vi "State_Modelling_2_state_sol..vi"() -> ()   [LabVIEW 2019]
uses:
  <vilib>/addons/Control Design/_Model Construction/NI_LinSys_Model Creation.lvlib
  <vilib>/addons/Control Design/_Model Construction/Model Creation.llb/Model Creation SubVI/cd_Create State Space Model.vi
  <vilib>/addons/Control Design/_State-Space Analysis/NI_CD_State-Space Analysis.lvlib
  <vilib>/addons/Control Design/_Utility/NI_CD_Model Viewer.lvlib
  <vilib>/addons/Control Design/_Utility/Model Viewer.llb/Model Viewer SubVI/cd_Draw State-Space Equation (SS).vi
  <vilib>/addons/Control Design/_Dynamic Analysis/NI_CD_Dynamic Analysis.lvlib
  <vilib>/addons/Control Design/_Dynamic Analysis/Dynamic Analysis.llb/Dynamic Analysis subVI/cd_Pole-Zero Map (State-Space).vi
  <vilib>/addons/Control Design/_Time Response Analysis/NI_CD_Time Response.lvlib
  <vilib>/addons/Control Design/_Time Response Analysis/Time Response.llb/Time Response subVI/cd_Initial Response (State-Space).vi
  <vilib>/addons/Control Design/_State Feedback Control/NI_CD_State Feedback Control.lvlib
  <vilib>/Analysis/NI_AALBase.lvlib
  <vilib>/Analysis/baseanly.llb/Real A x B.vi
  <vilib>/Analysis/Matrix/NI_Matrix.lvlib
  <vilib>/Analysis/Matrix/Numeric/Subtract/Subtract - RM,RM.vi
  <vilib>/addons/Control Design/_Dynamic Analysis/Dynamic Analysis.llb/Dynamic Analysis subVI/cd_Root Locus (State-Space).vi
panel:
  in  "Compenstaed Root Locus Gain":dbl[](array[numeric])=[1e-18] format="%.2f"
  out "Compensated Root Locus":cluster{dbl[], dbl[]}[](graph)=[{[-5.0, -5.0], [1.0323827311807139e-07, -1.0323827311807139e-07]}, {[-4.999999999999999, -4.999999999999999], [1.0323827311807139e-07, -1.0323827311807139e-07]}, {[], []}, {[-4.999999999999999], [0.0]}, {array[592 elements], [1.0323827311807139e-07, 5.960464477539063e-08, 5.960464477539063e-08, 5.960464477539063e-08, 5.960464477539063e-08, 5.960464477539063e-08, 5.960464477539063e-08, 5.960464477539063e-08, 5.960464477539063e-08, 5.960464477539063e-08, 5.960464477539063e-08, 0.0, 0.0, 0.0, 0.0, 0.0, 0.0, 0.0, 0.0, 0.0, 0.0, 0.0, 0.0, 0.0, 0.0, 0.0, 0.0, 0.0, 0.0, 0.0, 0.0, 0.0, 0.0, 0.0, 0.0, 0.0, 0.0, 0.0, 0.0, 0.0, 0.0, 0.0, 0.0, 0.0, 0.0, 0.0, 0.0, 0.0, 0.0, 0.0, 0.0, 0.0, 0.0, 0.0, 0.0, 0.0, 0.0, 0.0, 0.0, 0.0, 0.0, 0.0, 0.0, 0.0, 0.0, 0.0, 0.0, 0.0, 0.0, 0.0, 0.0, 0.0, 0.0, 0.0, 0.0, 0.0, 0.0, 0.0, 0.0, 0.0, 0.0, 0.0, 0.0, 0.0, 0.0, 0.0, 0.0, 0.0, 0.0, 0.0, 0.0, 0.0, 0.0, 0.0, 0.0, 0.0, 0.0, 0.0, 0.0, 0.0, 0.0, 0.0, 0.0, 0.0, 0.0, 0.0, 0.0, 0.0, 0.0, 0.0, 0.0, 0.0, 0.0, 0.0, 0.0, 0.0, 0.0, 0.0, 0.0, 0.0, 0.0, 0.0, 0.0, 0.0, 0.0, 0.0, 0.0, 0.0, 0.0, 0.0, 0.0, 0.0, 0.0, 0.0, 0.0, 0.0, 0.0, 0.0, 0.0, 0.0, 0.0, 0.0, 0.0, 0.0, 0.0, 0.0, 0.0, 0.0, 0.0, 0.0, 0.0, 0.0, 0.0, 0.0, 0.0, 0.0, 0.0, 0.0, 0.0, 0.0, 0.0, 0.0, 0.0, 0.0, 0.0, 0.0, 0.0, 0.0, 0.0, 0.0, 0.0, 0.0, 0.0, 0.0, 0.0, 0.0, 0.0, 0.0, 0.0, 0.0, 0.0, 0.0, 0.0, 0.0, 0.0, 0.0, 0.0, 0.0, 0.0, 0.0, 0.0, 0.0, 0.0, 0.0, 0.0, 0.0, 0.0, 0.0, 0.0, 0.0, 0.0, 0.0, 0.0, 0.0, 0.0, 0.0, 0.0, 0.0, 0.0, 0.0, 0.0, 0.0, 0.0, 0.0, 0.0, 0.0, 0.0, 0.0, 0.0, 0.0, 0.0, 0.0, 0.0, 0.0, 0.0, 0.0, 0.0, 0.0, 0.0, 0.0, 0.0, 0.0, 0.0, 0.0, 0.0, 0.0, 0.0, 0.0, 0.0, 0.0, 0.0, 0.0, 0.0, 0.0, 0.0, 0.0, 0.0, 0.0, 0.0, 0.0, 0.0, 0.0, 0.0, 0.0, 0.0, 0.0, 0.0, 0.0, 0.0, 0.0, 0.0, 0.0, 0.0, 0.0, 0.0, 0.0, 0.0, 0.0, 0.0, 0.0, 0.0, 0.0, 0.0, 0.0, 0.0, 0.0, 0.0, 0.0, 0.0, 0.0, 0.0, 0.0, 0.0, 0.0, 0.0, 0.0, 0.0, 0.0, 0.0, 0.0, 0.0, 0.0, 0.0, 0.0, 0.0, 0.0, 0.0, 0.0, 0.0, 0.0, 0.0, 0.0, 0.0, 0.0, 0.0, 0.0, 0.0, 0.0, 0.0, 0.0, 0.0, 0.0, 0.0, 0.0, 0.0, 0.0, 0.0, 0.0, 0.0, 0.0, 0.0, 0.0, 0.0, nan, nan, nan, nan, nan, nan, nan, nan, nan, nan, nan, nan, nan, nan, nan, nan, nan, nan, nan, nan, nan, nan, nan, nan, nan, nan, nan, nan, nan, nan, nan, nan, nan, nan, nan, nan, nan, nan, nan, nan, nan, nan, nan, nan, nan, nan, nan, nan, nan, nan, nan, nan, nan, nan, nan, nan, nan, nan, nan, nan, nan, nan, nan, nan, nan, nan, nan, nan, nan, nan, nan, nan, nan, nan, nan, nan, nan, nan, nan, nan, nan, nan, nan, nan, nan, nan, nan, nan, nan, nan, nan, nan, nan, nan, nan, nan, nan, nan, nan, nan, nan, nan, nan, nan, nan, nan, nan, nan, nan, nan, nan, nan, nan, nan, nan, nan, nan, nan, nan, nan, nan, nan, nan, nan, nan, nan, nan, nan, nan, nan, nan, nan, nan, nan, nan, nan, nan, nan, nan, nan, nan, nan, nan, nan, nan, nan, nan, nan, nan, nan, nan, nan, nan, nan, nan, nan, nan, nan, nan, nan, nan, nan, nan, nan, nan, nan, nan, nan, nan, nan, nan, nan, nan, nan, nan, nan, nan, nan, nan, nan, nan, nan, nan, nan, nan, nan, nan, nan, nan, nan, nan, nan, nan, nan, nan, nan, nan, nan, nan, nan, nan, nan, nan, nan, nan, nan, nan, nan, nan, nan, nan, nan, nan, nan, nan, nan, nan, nan, nan, nan, nan, nan, nan, nan, nan, nan, nan, nan, nan, nan, nan, nan, nan, nan, nan, nan, nan, nan, nan, nan, nan, nan, nan, nan, nan, nan, nan, nan, nan, nan, nan, nan, nan, nan, nan, nan, nan, nan, nan, nan, nan, nan, nan, nan, nan, nan, nan, nan, nan]}, {array[592 elements], [-1.0323827311807139e-07, -5.960464477539063e-08, -5.960464477539063e-08, -5.960464477539063e-08, -5.960464477539063e-08, -5.960464477539063e-08, -5.960464477539063e-08, -5.960464477539063e-08, -5.960464477539063e-08, -5.960464477539063e-08, -5.960464477539063e-08, 0.0, 0.0, 0.0, 0.0, 0.0, 0.0, 0.0, 0.0, 0.0, 0.0, 0.0, 0.0, 0.0, 0.0, 0.0, 0.0, 0.0, 0.0, 0.0, 0.0, 0.0, 0.0, 0.0, 0.0, 0.0, 0.0, 0.0, 0.0, 0.0, 0.0, 0.0, 0.0, 0.0, 0.0, 0.0, 0.0, 0.0, 0.0, 0.0, 0.0, 0.0, 0.0, 0.0, 0.0, 0.0, 0.0, 0.0, 0.0, 0.0, 0.0, 0.0, 0.0, 0.0, 0.0, 0.0, 0.0, 0.0, 0.0, 0.0, 0.0, 0.0, 0.0, 0.0, 0.0, 0.0, 0.0, 0.0, 0.0, 0.0, 0.0, 0.0, 0.0, 0.0, 0.0, 0.0, 0.0, 0.0, 0.0, 0.0, 0.0, 0.0, 0.0, 0.0, 0.0, 0.0, 0.0, 0.0, 0.0, 0.0, 0.0, 0.0, 0.0, 0.0, 0.0, 0.0, 0.0, 0.0, 0.0, 0.0, 0.0, 0.0, 0.0, 0.0, 0.0, 0.0, 0.0, 0.0, 0.0, 0.0, 0.0, 0.0, 0.0, 0.0, 0.0, 0.0, 0.0, 0.0, 0.0, 0.0, 0.0, 0.0, 0.0, 0.0, 0.0, 0.0, 0.0, 0.0, 0.0, 0.0, 0.0, 0.0, 0.0, 0.0, 0.0, 0.0, 0.0, 0.0, 0.0, 0.0, 0.0, 0.0, 0.0, 0.0, 0.0, 0.0, 0.0, 0.0, 0.0, 0.0, 0.0, 0.0, 0.0, 0.0, 0.0, 0.0, 0.0, 0.0, 0.0, 0.0, 0.0, 0.0, 0.0, 0.0, 0.0, 0.0, 0.0, 0.0, 0.0, 0.0, 0.0, 0.0, 0.0, 0.0, 0.0, 0.0, 0.0, 0.0, 0.0, 0.0, 0.0, 0.0, 0.0, 0.0, 0.0, 0.0, 0.0, 0.0, 0.0, 0.0, 0.0, 0.0, 0.0, 0.0, 0.0, 0.0, 0.0, 0.0, 0.0, 0.0, 0.0, 0.0, 0.0, 0.0, 0.0, 0.0, 0.0, 0.0, 0.0, 0.0, 0.0, 0.0, 0.0, 0.0, 0.0, 0.0, 0.0, 0.0, 0.0, 0.0, 0.0, 0.0, 0.0, 0.0, 0.0, 0.0, 0.0, 0.0, 0.0, 0.0, 0.0, 0.0, 0.0, 0.0, 0.0, 0.0, 0.0, 0.0, 0.0, 0.0, 0.0, 0.0, 0.0, 0.0, 0.0, 0.0, 0.0, 0.0, 0.0, 0.0, 0.0, 0.0, 0.0, 0.0, 0.0, 0.0, 0.0, 0.0, 0.0, 0.0, 0.0, 0.0, 0.0, 0.0, 0.0, 0.0, 0.0, 0.0, 0.0, 0.0, 0.0, 0.0, 0.0, 0.0, 0.0, 0.0, 0.0, 0.0, 0.0, 0.0, 0.0, 0.0, 0.0, 0.0, 0.0, 0.0, 0.0, 0.0, 0.0, 0.0, 0.0, 0.0, 0.0, 0.0, 0.0, 0.0, 0.0, 0.0, 0.0, 0.0, 0.0, 0.0, 0.0, 0.0, 0.0, 0.0, 0.0, 0.0, 0.0, 0.0, 0.0, 0.0, 0.0, 0.0, 0.0, 0.0, 0.0, 0.0, 0.0, 0.0, 0.0, 0.0, 0.0, 0.0, 0.0, 0.0, 0.0, 0.0, 0.0, 0.0, 0.0, 0.0, 0.0, 0.0, 0.0, 0.0, 0.0, 0.0, 0.0, 0.0, 0.0, 0.0, 0.0, 0.0, 0.0, 0.0, 0.0, 0.0, 0.0, 0.0, 0.0, 0.0, 0.0, 0.0, 0.0, 0.0, 0.0, 0.0, 0.0, 0.0, 0.0, 0.0, 0.0, 0.0, 0.0, 0.0, 0.0, 0.0, 0.0, 0.0, 0.0, 0.0, 0.0, 0.0, 0.0, 0.0, 0.0, 0.0, 0.0, 0.0, 0.0, 0.0, 0.0, 0.0, 0.0, 0.0, 0.0, 0.0, 0.0, 0.0, 0.0, 0.0, 0.0, 0.0, 0.0, 0.0, 0.0, 0.0, 0.0, 0.0, 0.0, 0.0, 0.0, 0.0, 0.0, 0.0, 0.0, 0.0, 0.0, 0.0, 0.0, 0.0, 0.0, 0.0, 0.0, 0.0, 0.0, 0.0, 0.0, 0.0, 0.0, 0.0, 0.0, 0.0, 0.0, 0.0, 0.0, 0.0, 0.0, 0.0, 0.0, 0.0, nan, nan, nan, nan, nan, nan, nan, nan, nan, nan, nan, nan, nan, nan, nan, nan, nan, nan, nan, nan, nan, nan, nan, nan, nan, nan, nan, nan, nan, nan, nan, nan, nan, nan, nan, nan, nan, nan, nan, nan, nan, nan, nan, nan, nan, nan, nan, nan, nan, nan, nan, nan, nan, nan, nan, nan, nan, nan, nan, nan, nan, nan, nan, nan, nan, nan, nan, nan, nan, nan, nan, nan, nan, nan, nan, nan, nan, nan, nan, nan, nan, nan, nan, nan, nan, nan, nan, nan, nan, nan, nan, nan, nan, nan, nan, nan, nan, nan, nan, nan, nan, nan, nan, nan, nan, nan, nan, nan, nan, nan, nan, nan, nan, nan, nan, nan, nan, nan, nan, nan, nan, nan, nan, nan, nan, nan, nan, nan, nan, nan, nan, nan, nan, nan, nan, nan, nan, nan, nan, nan, nan, nan, nan, nan, nan, nan, nan, nan, nan, nan]}]
  out "Root Locus Graph":cluster{dbl[], dbl[]}[](graph)=[{[-1.1574212961095778e-15, -1.1574212961095778e-15], [-18.902124219251128, 18.902124219251128]}, {[-0.0, -0.0], [18.902124219251128, -18.902124219251128]}, {[], []}, {[0.0], [0.0]}, {array[574 elements], array[574 elements]}, {array[574 elements], array[574 elements]}]
  in  "Root Locus Gain":dbl[](array[numeric])=[0.0] format="%.2f"
  in  "Desired Poles":cdb[](array[numeric])=[-5.0+0.0i, -5.0+0.0i] format="%.2f"
  in  "D":dbl[][](array[numeric])=[[0.0]] format="%#.5g"
  in  "C":dbl[][](array[numeric])=[[1.0, 0.0]] format="%#.5g"
  in  "B":dbl[][](array[numeric])=[[0.0], [-36.421]] format="%#.5g"
  in  "A":dbl[][](array[numeric])=[[0.0, 1.0], [-357.2903, 0.0]] format="%#.5g"
  in  "Initial Conditions":dbl[](array[numeric])=[0.572, 0.0] format="%.3f"
  out "State Trajectory Graph Compensated":cluster{"time":dbl[], dbl[]}[](graph)=[{"time"=[0.0, 0.04000000000000001, 0.08000000000000002, 0.12000000000000002, 0.16000000000000003, 0.20000000000000004, 0.24000000000000005, 0.28, 0.32000000000000006, 0.3600000000000001, 0.4000000000000001, 0.44000000000000006, 0.4800000000000001, 0.5200000000000001, 0.56, 0.6000000000000001, 0.6400000000000001, 0.6800000000000002, 0.7200000000000002, 0.7600000000000001, 0.8000000000000002, 0.8400000000000002, 0.8800000000000001, 0.9200000000000002, 0.9600000000000002, 1.0000000000000002, 1.0400000000000003, 1.0800000000000003, 1.12, 1.1600000000000001, 1.2000000000000002, 1.2400000000000002, 1.2800000000000002, 1.3200000000000003, 1.3600000000000003, 1.4000000000000004, 1.4400000000000004, 1.4800000000000002, 1.5200000000000002, 1.5600000000000003, 1.6000000000000003], [0.572, 0.5619767889127265, 0.5367922928653396, 0.5022724093532525, 0.46262910145509073, 0.4208540807001293, 0.3790227962703144, 0.3385283120990366, 0.30026050156165074, 0.2647426993756922, 0.23223534603402665, 0.20281410106641523, 0.17642827555724877, 0.1529441522589557, 0.13217675212217317, 0.11391281242567214, 0.09792711883762648, 0.08399384583614819, 0.07189417850331574, 0.06142119120828786, 0.0523827272217794, 0.044602843694828566, 0.03792224749259751, 0.03219804025721003, 0.027303008809828617, 0.023124634100861116, 0.01956394406178582, 0.016534299514716293, 0.013960175102466216, 0.01177597693761364, 0.009924923715371986, 0.008358007132520252, 0.007033039625890542, 0.005913791932828125, 0.004969219199624306, 0.004172771874377408, 0.003501786075609926, 0.0029369472666753264, 0.002461820691381014, 0.0020624419901926214, 0.0017269616084421026]}, {"time"=[0.0, 0.04000000000000001, 0.08000000000000002, 0.12000000000000002, 0.16000000000000003, 0.20000000000000004, 0.24000000000000005, 0.28, 0.32000000000000006, 0.3600000000000001, 0.4000000000000001, 0.44000000000000006, 0.4800000000000001, 0.5200000000000001, 0.56, 0.6000000000000001, 0.6400000000000001, 0.6800000000000002, 0.7200000000000002, 0.7600000000000001, 0.8000000000000002, 0.8400000000000002, 0.8800000000000001, 0.9200000000000002, 0.9600000000000002, 1.0000000000000002, 1.0400000000000003, 1.0800000000000003, 1.12, 1.1600000000000001, 1.2000000000000002, 1.2400000000000002, 1.2800000000000002, 1.3200000000000003, 1.3600000000000003, 1.4000000000000004, 1.4400000000000004, 1.4800000000000002, 1.5200000000000002, 1.5600000000000003, 1.6000000000000003], [0.0, -0.46831399076060565, -0.7668461326647711, -0.9417607675373487, -1.028064669900202, -1.0521352017503238, -1.0336985352826762, -0.9873742436221906, -0.9238784663435413, -0.8509586765647255, -0.7741178201134225, -0.6971734724158027, -0.6226880313785255, -0.5522983276017848, -0.4869669815027436, -0.42717304659627087, -0.37305569081000595, -0.32452167709420926, -0.28132504631732275, -0.24312554853280632, -0.20953090888711776, -0.18012686876757705, -0.15449804534021222, -0.13224195105639847, -0.11297796748894612, -0.09635264208692143, -0.08204234606555352, -0.06975407607770943, -0.059224985283190076, -0.05022107811629353, -0.04253538735159428, -0.03598586404279558, -0.030413144328175358, -0.02567830707675374, -0.02166069907528547, -0.018255876950401186, -0.01537369496609238, -0.012936553436546098, -0.010877812357264961, -0.00914036791108095, -0.007675384926409356]}]
  out "Comp poles":cdb[](array[numeric])=[-4.999999999999999+9.425385918369788e-08i, -4.999999999999999-9.425385918369788e-08i] caption="Poles Compensated" format="%.4f"
  out "Pole-Zero Map Comp":cluster{dbl[], dbl[]}[](graph)=[{[-4.999999999999999, -4.999999999999999], [9.425385918369788e-08, -9.425385918369788e-08]}, {[], []}] caption="Pole-Zero Map Compensated"
  out "Actual Poles":cdb[](array[numeric])=[-4.999999999999999+9.425385918369788e-08i, -4.999999999999999-9.425385918369788e-08i] format="%.2f"
  out "Gain":dbl[][](array[numeric])=[[9.123590785535818, -0.27456687076137387]] format="%.2f"
  out "State Trajectory Graph":cluster{"time":dbl[], dbl[]}[](graph)
  out "Uncomp Poles":cdb[](array[numeric])=[0.0+18.902124219251128i, 0.0-18.902124219251128i] caption="Poles Uncompensated" format="%.4f"
  out "Pole-Zero Map":cluster{dbl[], dbl[]}[](graph)=[{[0.0, 0.0], [18.902124219251128, -18.902124219251128]}, {[], []}]
  out "Equation":picture
  out "Transformation Matrix (T)":dbl[][](array[numeric])=[[18.9285577897525, 0.0], [-0.0, 1.0013984444390887]] format="%.2f"
  in  "Form Type":u16(ring) items=["Modal"=0, "Companion"=5, "Controllability"=1, "Controller Companion"=2, "Observability"=3, "Observer Companion"=4]
  out "Is Controllable?":bool=TRUE
  out "Controllability Matrix":dbl[][](array[numeric])=[[0.0, -36.421], [-36.421, 0.0]] format="%.2f"
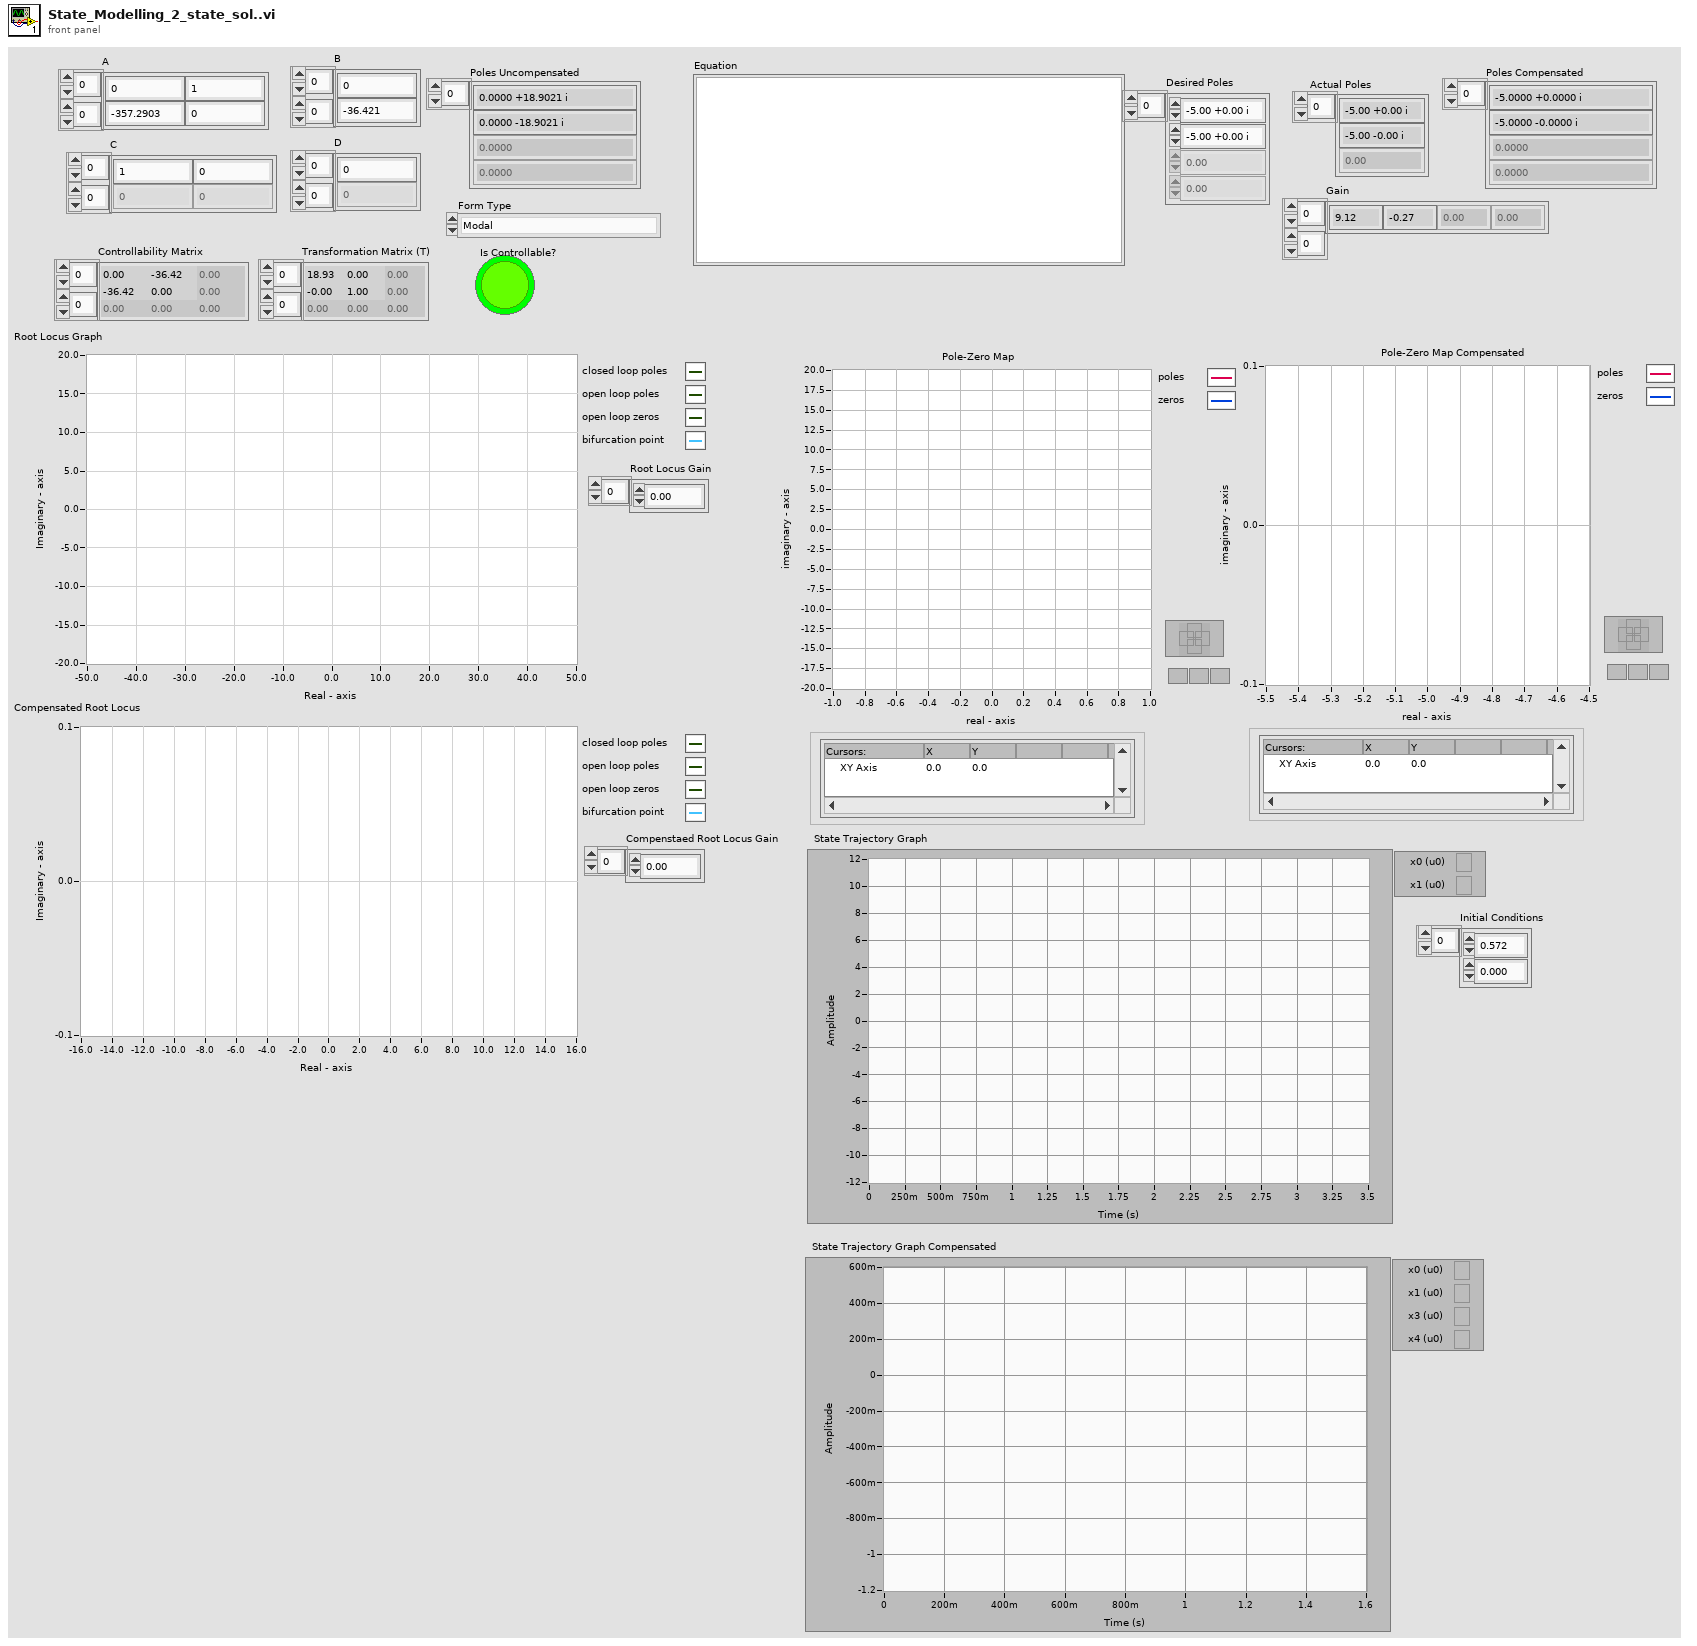
[diagram p1: front panel]
types:
  T1 = typedef "NI_LinSys_Model Typedefs.lvlib/CD State Space Model (MIMO).ctl" = cluster{"properties":T2, "A":dbl[][], "B":dbl[][], "C":dbl[][], "D":dbl[][], "StateNames":string[], "Transport Delay":dbl[][]}
  T2 = typedef "NI_LinSys_Model Typedefs.lvlib/CD General Elements.ctl" = cluster{"Model name":string, "Input names":string[], "Output names":string[], "Input Delays":dbl[], "Output Delays":dbl[], "Sampling Time":dbl, "Notes":string}
  T3 = typedef "NI_Matrix.lvlib/RealMatrix.ctl" = dbl[][]
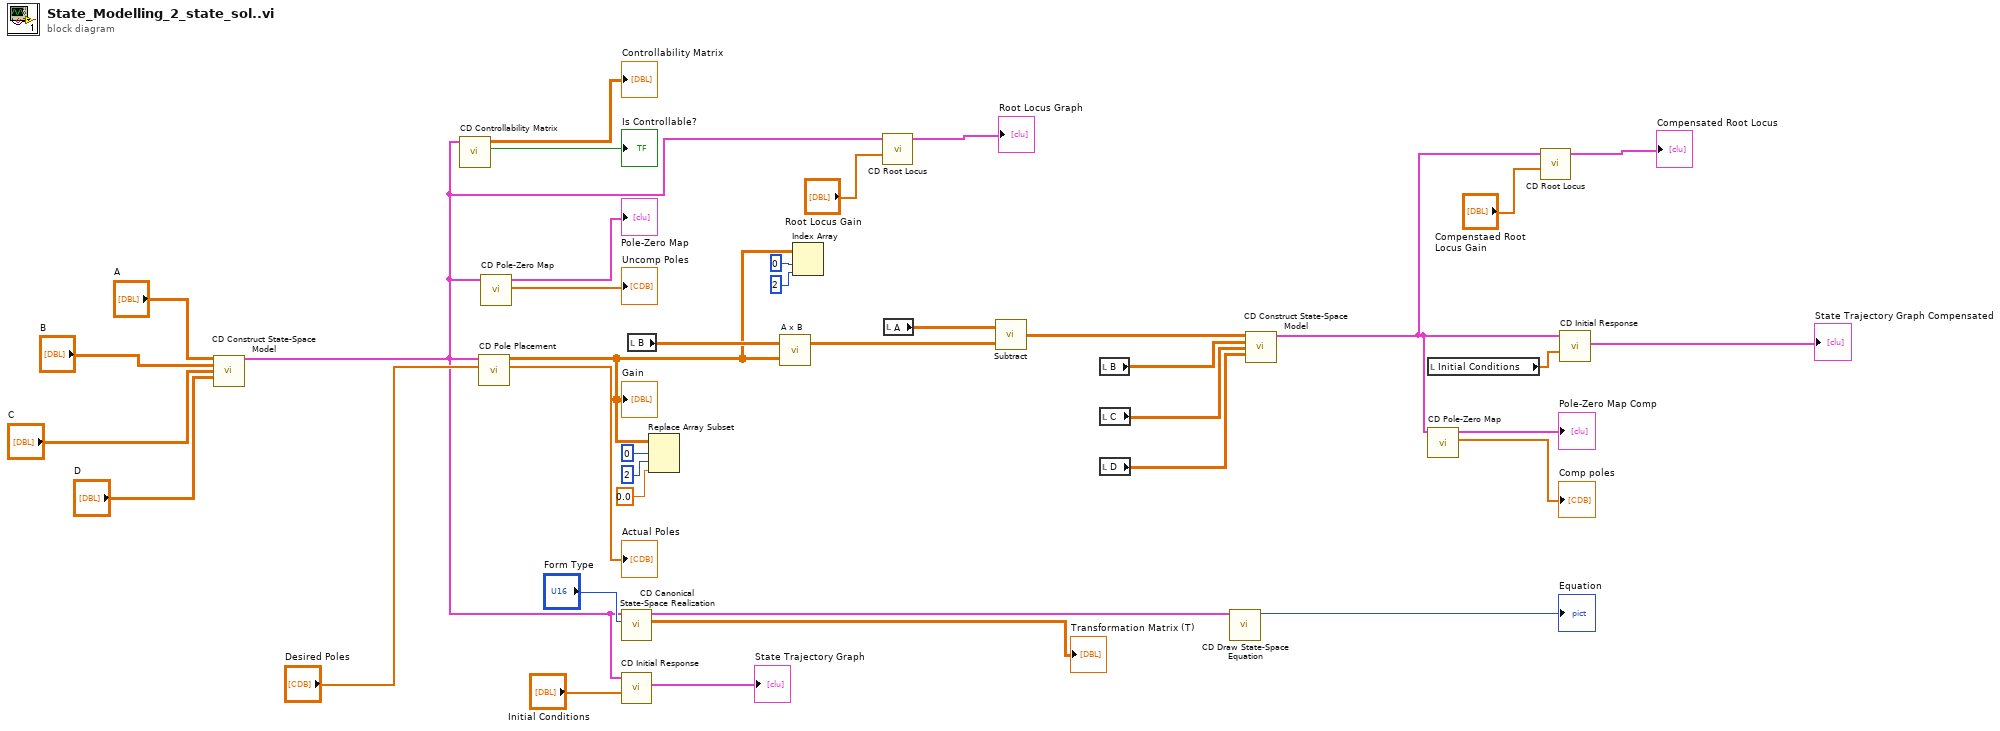
[diagram p0: block diagram]
diagram:
  n1 = call-poly <vilib>:"CD Construct State-Space Model.vi"("A"="A", "B"="B", "C"="C", "D"="D") -> ("State-Space Model"=w6:T1)  [unwired: 10 in, 1 out]
  n2 = call <vilib>:"CD Controllability Matrix.vi"("State-Space Model"=w6) -> ("Is Controllable?"=→"Is Controllable?":bool, "Controllability Matrix"=→"Controllability Matrix":dbl[][])  [unwired: 7 in, 2 out]
  n3 = call <vilib>:"CD Pole Placement.vi"("Poles"="Desired Poles", "State-Space Model"=w6) -> ("Actual Poles"=→"Actual Poles":cdb[], "Gain"=w8:dbl[][])  [unwired: 7 in, 1 out]
  "Gain" <- w8
  n4 = call-poly <vilib>:"CD Pole-Zero Map.vi"("State-Space Model"=w6) -> ("Poles"=→"Uncomp Poles":cdb[], "Pole-Zero Map"=→"Pole-Zero Map":cluster{dbl[], dbl[]}[])  [unwired: 7 in, 2 out]
  n5 = call <vilib>:"CD Canonical State-Space Realization.vi"("Form Type"="Form Type", "State-Space Model"=w6) -> ("Transformation Matrix (T)"=→"Transformation Matrix (T)":dbl[][], "Transformed Model"=w35:T1)  [unwired: 7 in, 1 out]
  n6 = call-poly <vilib>:"CD Initial Response.vi"("Initial Conditions"="Initial Conditions", "State-Space Model"=w6) -> ("State Trajectory Graph"=→"State Trajectory Graph":cluster{"time":dbl[], dbl[]}[])  [unwired: 6 in, 3 out]
  n7 = local read "B"() -> (w14:dbl[][])
  n8 = Replace Array Subset(array=w8, new element=0.0 ("new element/subarray"), index (row)=0, index (col)=2 ("disabled index (col)")) -> ()  [unwired: 1 out]
  n9 = call-poly <vilib>:"A x B.vi"("B"=w8, "A"=w14) -> ("A x B"=w28:T3)  [unwired: 1 out]
  n10 = Index Array(array=w8, index (row)=0, index (col)=2 ("disabled index (col)")) -> ()  [unwired: 1 out]
  n11 = call-poly <vilib>:"CD Root Locus.vi"("Gain"="Root Locus Gain", "State-Space Model"=w6) -> ("Root Locus Graph"=→"Root Locus Graph":cluster{dbl[], dbl[]}[])  [unwired: 6 in, 3 out]
  n12 = local read "A"() -> (w18:dbl[][])
  n13 = call-poly <vilib>:"Subtract.vi"("Real Matrix B"=w28, "Real Matrix A"=w18) -> ("A - B"=w26:T3)
  n14 = local read "B"() -> (w17:dbl[][])
  n15 = local read "C"() -> (w16:dbl[][])
  n16 = local read "D"() -> (w15:dbl[][])
  n17 = call-poly <vilib>:"CD Draw State-Space Equation.vi"("State-Space Model"=w35) -> ("Equation"=→"Equation":picture)  [unwired: 8 in, 2 out]
  n18 = call-poly <vilib>:"CD Construct State-Space Model.vi"("A"=w26, "B"=w17, "C"=w16, "D"=w15) -> ("State-Space Model"=w1:T1)  [unwired: 10 in, 1 out]
  n19 = local read "Initial Conditions"() -> (w19:dbl[])
  n20 = call-poly <vilib>:"CD Pole-Zero Map.vi"("State-Space Model"=w1) -> ("Poles"=→"Comp poles":cdb[], "Pole-Zero Map"=→"Pole-Zero Map Comp":cluster{dbl[], dbl[]}[])  [unwired: 7 in, 2 out]
  n21 = call-poly <vilib>:"CD Root Locus.vi"("Gain"="Compenstaed Root Locus Gain", "State-Space Model"=w1) -> ("Root Locus Graph"=→"Compensated Root Locus":cluster{dbl[], dbl[]}[])  [unwired: 6 in, 3 out]
  n22 = call-poly <vilib>:"CD Initial Response.vi"("Initial Conditions"=w19, "State-Space Model"=w1) -> ("State Trajectory Graph"=→"State Trajectory Graph Compensated":cluster{"time":dbl[], dbl[]}[])  [unwired: 6 in, 3 out]
